vi "XL320_Configure Safety Settings.vi"(0 "VISA resource name":refnum<visa-resource-name>, 5 "Motor ID (0)":u8, 7 "Alarm Settings":cluster{"LED Alarm":T1, "Shutdown Alarm":T1}, 9 "Safety Limits":T2={"Temperature Limit (C)"=65, "Low Voltage Limit (V)"=6.0, "High Voltage Limit (V)"=9.0, "Maximum Torque%"=100.0}, 11 "error in (no error)":errorcluster) -> (4 "VISA resource name out":refnum<visa-resource-name>, 15 "error out":errorcluster)   [LabVIEW 2017, in "Dynamixel XL320.lvlib"]
doc: "Sets limits for the temperature, voltage, and torque for the motor as well as the action to take for status errors for: temperature, overload, angle limit, checksum, etc."
uses:
  <instrlib>/Dynamixel XL320 (Drivers instrument)/Dynamixel XL320.lvlib
  <instrlib>/Dynamixel XL320 (Drivers instrument)/Public/Motor Operation/Low Level/XL320_Alarm Setting.ctl
panel:
  # "Ghislain REMY, IUT de Cachan, 2015 December 2015"
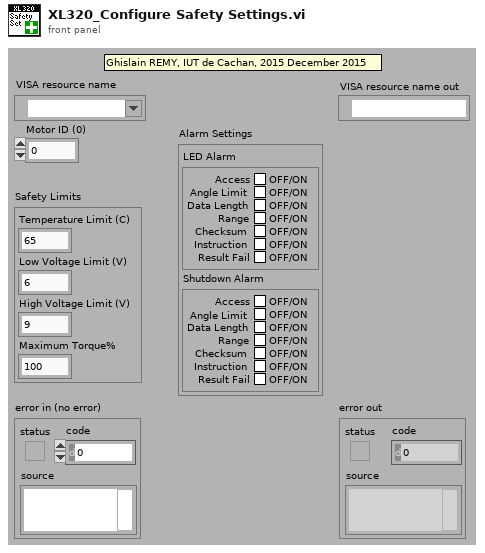
[diagram p1: front panel]
types:
  T1 = typedef "Dynamixel XL320.lvlib/XL320_Alarm Setting.ctl" = cluster{"Access":bool, "Angle Limit":bool, "Data Length":bool, "Range":bool, "Checksum":bool, "Instruction":bool, "Result Fail":bool}
  T2 = cluster{"Temperature Limit (C)":u8, "Low Voltage Limit (V)":dbl, "High Voltage Limit (V)":dbl, "Maximum Torque%":dbl}
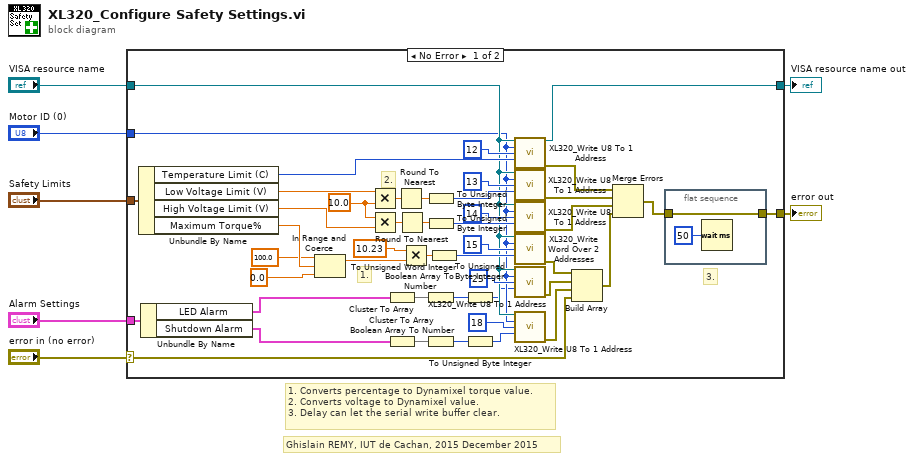
[diagram p0: block diagram]
diagram:
  # "Ghislain REMY, IUT de Cachan, 2015 December 2015"
  # "1. Converts percentage to Dynamixel torque value.\n2. Converts voltage to Dynamixel value.\n3. Delay can let the serial write buffer clear."
  n1 = case shown="No Error" "error in (no error)" {
    selector: "error in (no error)" -> [w38 w57]
    tunnel: "VISA resource name" -> [w15 w56]
    tunnel: "Motor ID (0)" -> [w14 _]
    tunnel: [w28 w56] -> w2
    tunnel: "Safety Limits" -> [w51 _]
    tunnel: [w34 w57] -> w3
    tunnel: "Alarm Settings" -> [w40 _]
    frame No Error {
      w47 = 10.0 ("y")
      # "3."
      # "2."
      # "1."
      n2 = Unbundle By Name(w51) -> ("Temperature Limit (C)"=w29:u8, "Low Voltage Limit (V)"=w49:dbl, "High Voltage Limit (V)"=w48:dbl, "Maximum Torque%"=w43:dbl)
      n3 = Unbundle By Name(w40) -> ("LED Alarm"=w37:T1, "Shutdown Alarm"=w36:T1)
      n4 = In Range and Coerce(upper limit=100.0, x=w43, lower limit=0.0) -> (coerced(x)=w33:dbl)  [unwired: 1 out]
      n5 = Multiply(x=w49, y=w47) -> (x*y=w46:dbl)
      n6 = Multiply(x=w47, y=w48) -> (x*y=w50:dbl)
      n7 = Cluster To Array(cluster=w37) -> (array=w42:bool[])
      n8 = Cluster To Array(cluster=w36) -> (array=w39:bool[])
      n9 = Round To Nearest(number=w46) -> (nearest integer value=w44:dbl)
      n10 = Round To Nearest(number=w50) -> (nearest integer value=w45:dbl)
      n11 = Multiply(x=10.23, y=w33) -> (x*y=w53:dbl)
      n12 = To Unsigned Byte Integer(number=w44) -> (unsigned 8bit integer=w25:u8)
      n13 = To Unsigned Byte Integer(number=w45) -> (unsigned 8bit integer=w21:u8)
      n14 = Boolean Array To Number(Boolean array=w42) -> (number=w9:u32)
      n15 = Boolean Array To Number(Boolean array=w39) -> (number=w11:u32)
      n16 = To Unsigned Word Integer(number=w53) -> (unsigned 16bit integer=w19:u16)
      n17 = To Unsigned Byte Integer(number=w9) -> (unsigned 8bit integer=w8:u8)
      n18 = To Unsigned Byte Integer(number=w11) -> (unsigned 8bit integer=w10:u8)
      n19 = call <instrlib>:"XL320_Write U8 To 1 Address.vi"("VISA resource name"=w15, "Motor ID (0)"=w14, "Address number (0)"=u16 12, "Parameter (0)"=w29) -> ("VISA resource name out"=w28:refnum<visa-resource-name>, "error out"=w27:errorcluster)  [unwired: 10 in]
      n20 = call <instrlib>:"XL320_Write U8 To 1 Address.vi"("VISA resource name"=w15, "Motor ID (0)"=w14, "Address number (0)"=u16 13, "Parameter (0)"=w25) -> ("error out"=w24:errorcluster)  [unwired: 10 in, 1 out]
      n21 = call <instrlib>:"XL320_Write U8 To 1 Address.vi"("VISA resource name"=w15, "Motor ID (0)"=w14, "Address number (0)"=u16 14, "Parameter (0)"=w21) -> ("error out"=w23:errorcluster)  [unwired: 10 in, 1 out]
      n22 = call <instrlib>:"XL320_Write Word Over 2 Addresses.vi"("VISA resource name"=w15, "Motor ID (0)"=w14, "Address number (0)"=u16 15, "Parameter (0)"=w19) -> ("error out"=w18:errorcluster)  [unwired: 10 in, 1 out]
      n23 = call <instrlib>:"XL320_Write U8 To 1 Address.vi"("VISA resource name"=w15, "Motor ID (0)"=w14, "Address number (0)"=u16 25, "Parameter (0)"=w8) -> ("error out"=w17:errorcluster)  [unwired: 10 in, 1 out]
      n24 = call <instrlib>:"XL320_Write U8 To 1 Address.vi"("VISA resource name"=w15, "Motor ID (0)"=w14, "Address number (0)"=u16 18, "Parameter (0)"=w10) -> ("error out"=w12:errorcluster)  [unwired: 10 in, 1 out]
      n25 = Build Array(w18, w17, w12, w38) -> (w41:errorcluster[])
      n26 = Merge Errors(w27, w24, w23, w41) -> (w35:errorcluster)
      n27 = flat-sequence {
        tunnel: w35 -> [w54]
        tunnel: [w54] -> w34
        frame #0 {
          n28 = Wait (ms)(milliseconds to wait=u32 50) -> ()  [unwired: 1 out]
        }
      }
    }
    frame Error {
    }
  }
  "VISA resource name out" <- w2
  "error out" <- w3
